vi "Generate digital signal.vi"(5 "number of channels":i32=2, 7 "interferrer channel":i32, 8 "phase":dbl, 9 "frequency":dbl=0.5, 10 "Output level in":dbl, 11 "Output level units":string) -> (2 "Output level out":dbl, 3 "Signal Properties":T1)   [LabVIEW 2021, in "Crosstalk_Audio DAC.lvlib"]
uses:
  Crosstalk_Audio DAC.lvlib
  <vilib>/PDM Acquisition Toolkit/host/Classes/Tasks/I2S Output/Control/SignalProperties.ctl
  <vilib>/PDM Acquisition Toolkit/host/Classes/Channels/I2S Ouput/Controls/GenerationChannelProperties.ctl
  <vilib>/PDM Acquisition Toolkit/host/Classes/Channels/I2S Ouput/I2S Output Channel.lvclass
  <vilib>/PDM Acquisition Toolkit/host/Classes/Tasks/I2S Output/I2S Output Task.lvclass
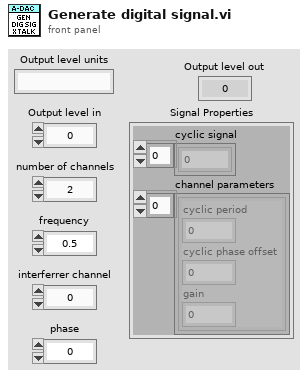
[diagram p1: front panel]
types:
  T1 = typedef "PDM Acquisition Class Library.lvlib/I2S Output Task.lvclass/SignalProperties.ctl" = cluster{"cyclic signal":dbl[], "channel parameters":T2[]}
  T2 = typedef "PDM Acquisition Class Library.lvlib/I2S Output Channel.lvclass/GenerationChannelProperties.ctl" = cluster{"cyclic period":dbl, "cyclic phase offset":dbl, "gain":dbl}
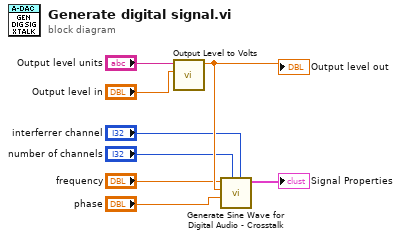
[diagram p0: block diagram]
diagram:
  n1 = call "Output Level to Volts.vi"("Output level in"="Output level in", "Output level units"="Output level units") -> ("Output level out"=w8:dbl)  [unwired: 9 in]
  "Output level out" <- w8
  n2 = call "Generate Sine Wave for Digital Audio - Crosstalk.vi"("interferrer channel"="interferrer channel", "number of channels"="number of channels", "phase"="phase", "gain"=w8, "frequency"="frequency") -> ("Signal Properties"=→"Signal Properties":T1)  [unwired: 6 in]
